vi "LINX - Servo 1 Channel.vi"() -> ()   [LabVIEW 2018]
doc: "This example demonstrates how to control a servo using LINX."
uses:
  <vilib>/MakerHub/LINX/Public/Peripherals/Digital/Digital Write 1 Chan.vi
  <vilib>/MakerHub/LINX/Public/Peripherals/Digital/Digital Write N Chans.vi
  <vilib>/MakerHub/LINX/Private/Local IO/LinxDigitalWrite.vi
  <vilib>/MakerHub/LINX/Public/Utilities/Check Channel.vi
  <vilib>/MakerHub/LINX/Public/Utilities/Open Serial.vi
  <vilib>/MakerHub/LINX/Public/Sensors/Motion/Servo/Servo Open One Channel.vi
  <vilib>/MakerHub/LINX/Private/Utilties/Generate Error.vi
  <vilib>/MakerHub/LINX/Public/Sensors/Motion/Servo/Servo Set Pulse Width One Channel.vi
  <vilib>/MakerHub/LINX/Public/Sensors/Motion/Servo/Servo Close One Channel.vi
  <vilib>/MakerHub/LINX/LMH-LINX.lvlib
  <vilib>/MakerHub/LINX/Public/Sensors/Motion/Servo/Servo.lvlib
panel:
  in  "Stop Button":bool
  in  "On/Off":bool
  in  "Servo Channel":u8=7
  in  "Serial Port":refnum<visa-resource-name>="COM5"
  # "Servo position \ncontrol"
  # "LINX Device Settings"
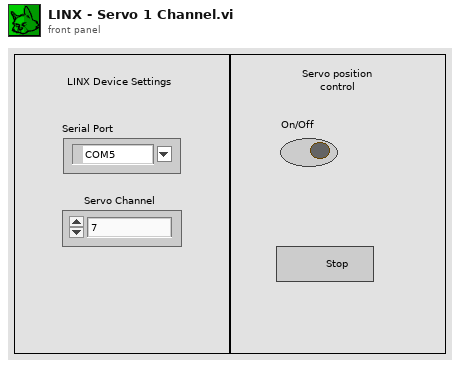
[diagram p1: front panel]
types:
  T1 = typedef "LMH-LINX.lvlib/LINX Ref.ctl" = cluster{"IO":T2, "Interface":T3, "LINX Device Config":T4}
  T2 = typedef "LMH-LINX.lvlib/Platform.ctl" = enum16{"Remote", "Local"}
  T3 = typedef "LMH-LINX.lvlib/Interface.ctl" = enum16{"Serial", "TCP"}
  T4 = typedef "LMH-LINX.lvlib/Device.lvlib/LINX Device Config.ctl" = cluster{"Interface":T3, "COM Port":refnum<visa-resource-name>, "TCP Configuration":T5, "Device Family":u8, "Device ID":u8, "Device Name":string, "TCP Ref":refnum<k5>, "Channels":T6}
  T5 = typedef "LMH-LINX.lvlib/Device.lvlib/TCP Config.ctl" = cluster{"IP Address":string, "Port":u16}
  T6 = typedef "LMH-LINX.lvlib/Channels.ctl" = cluster{"DI":u8[], "DO":u8[], "AI":u8[], "AO":u8[], "PWM":u8[], "QE":u8[], "UART":u8[], "I2C 2":u8[], "SPI":u8[], "CAN":u8[], "Servo":u8[], "AI Ref (V)":dbl, "AI Resolution (Bits)":u8, "AO Ref (V)":dbl, "AO Resolution (Bits)":u8}
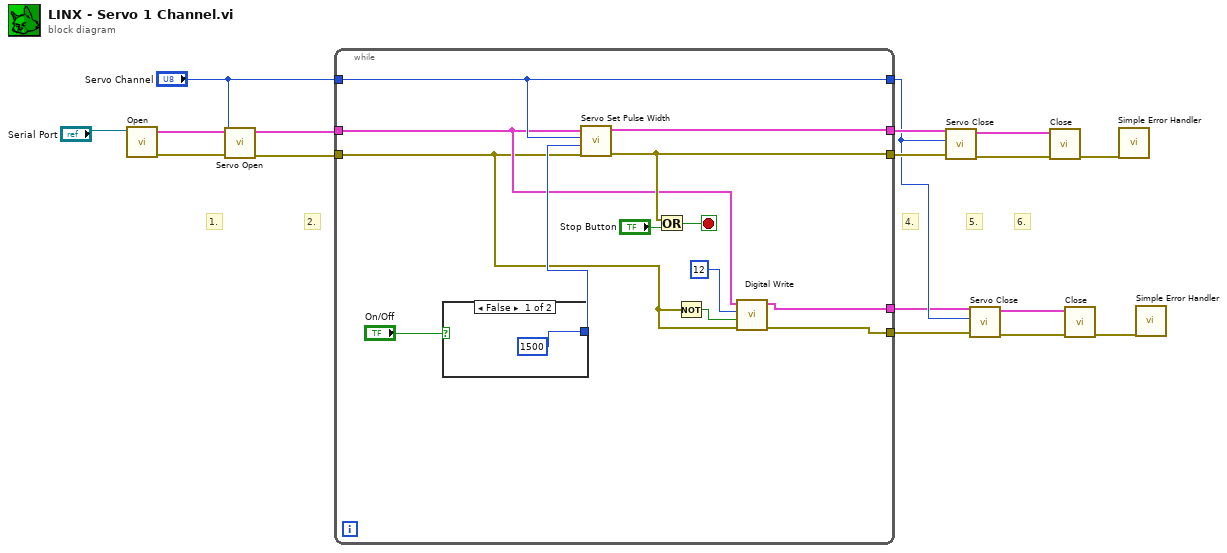
[diagram p0: block diagram]
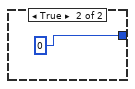
[diagram p2: hidden frame]
diagram:
  # "6."
  # "5."
  # "4."
  # "2."
  # "1."
  n1 = call-poly <vilib>:"Open.vi"("Serial Port"="Serial Port") -> ("Error Out"=w16:errorcluster, "LINX Resource"=w15:T1)  [unwired: 8 in, 1 out]
  n2 = call-poly <vilib>:"Servo Open.vi"("Error In"=w16, "Servo Channel"="Servo Channel", "LINX Resource"=w15) -> ("Error Out"=w14:errorcluster, "LINX Resource"=w13:T1)  [unwired: 7 in]
  n3 = while {
    tunnel: "Servo Channel" -> [w26]
    tunnel: [w26] -> w3
    tunnel: w13 -> [w22]
    tunnel: [w27] -> w10
    tunnel: w14 -> [w19]
    tunnel: [w28] -> w7
    tunnel: [w23] -> w2
    tunnel: [w21] -> w1
    stop <- w30 stop-if-true
    n4 = case shown="False" "On/Off" {
      tunnel: [1500 0] -> w24
      frame False {
      }
      frame True {
      }
    }
    n5 = call-poly <vilib>:"Servo Set Pulse Width.vi"("Error In"=w19, "Pulse Width (uS)"=w24, "Servo Channel"=w26, "LINX Resource"=w22) -> ("Error Out"=w28:errorcluster, "LINX Resource"=w27:T1)  [unwired: 6 in]
    n6 = Or(x=w28, y="Stop Button") -> (x .or. y?=w30:bool)
    n7 = Not(x=w19) -> (.not. x?=w18:bool)
    n8 = call-poly <vilib>:"Digital Write.vi"("Error In"=w19, "Output Value"=w18, "DO Channel"=u8 12, "LINX Resource"=w22) -> ("Error Out"=w21:errorcluster, "LINX Resource"=w23:T1)  [unwired: 6 in]
  }
  n9 = call-poly <vilib>:"Servo Close.vi"("Error In"=w7, "Servo Channel"=w3, "LINX Resource"=w10) -> ("Error Out"=w8:errorcluster, "LINX Resource"=w9:T1)  [unwired: 7 in]
  n10 = call-poly <vilib>:"Servo Close.vi"("Error In"=w1, "Servo Channel"=w3, "LINX Resource"=w2) -> ("Error Out"=w4:errorcluster, "LINX Resource"=w5:T1)  [unwired: 7 in]
  n11 = call <vilib>:"Close.vi"("Error In"=w8, "LINX Resource"=w9) -> ("Error Out"=w11:errorcluster)  [unwired: 9 in]
  n12 = call <vilib>:"Close.vi"("Error In"=w4, "LINX Resource"=w5) -> ("Error Out"=w6:errorcluster)  [unwired: 9 in]
  n13 = call <vilib>:"Simple Error Handler.vi"("error in (no error)"=w11) -> ()  [unwired: 4 in, 5 out]
  n14 = call <vilib>:"Simple Error Handler.vi"("error in (no error)"=w6) -> ()  [unwired: 4 in, 5 out]
